vi "9205_Initialize.vi"(7 "Module Model":T1=enum."NI 9205", 8 "error in (no error)":errorcluster, 9 "Slot Settings":T2, 11 "9205 in":refnum<class "9205.lvclass">) -> (0 "error out":errorcluster, 3 "9205 out":refnum<class "9205.lvclass">)   [LabVIEW 2017, in "Modules.lvlib" / "9205.lvclass"]
uses:
  9205.lvclass
  RSI Module/Slot Settings.ctl
  C:/Users/dbuck/Documents/GitHub/Scan-Engine-Custom-Device-Classes/Source/RSI Module/RSI Module.lvclass
  RSI Module/Module Models.ctl
  RSI Module/Channels.ctl
  RSI Module/Channel Type.ctl
  Channel Settings.ctl
  Range.ctl
  Terminal mode.ctl
  9205.lvclass/9205.ctl
  RSI Module/RSI Module.lvclass
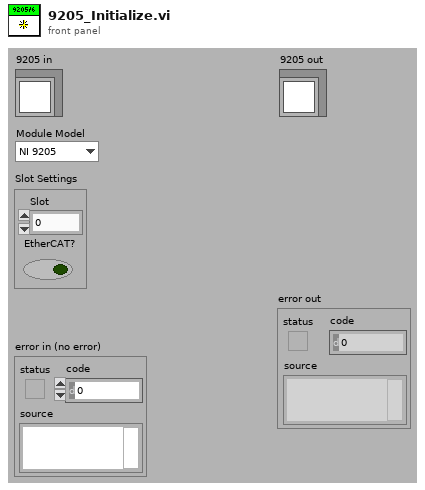
[diagram p1: front panel]
types:
  T1 = typedef "Modules.lvlib/RSI Module.lvclass/Module Models.ctl" = enum16{"Empty", "NI 9201", "NI 9203", "NI 9205", "NI 9206", "NI 9207", "NI 9208", "NI 9211", "NI 9212", "NI 9213", "NI 9214", "NI 9215", "NI 9217", "NI 9219", "NI 9220", "NI 9221", "NI 9222", "NI 9223", "NI 9225", "NI 9227", "NI 9229", "NI 9233", "NI 9234", "NI 9235", "NI 9236", "NI 9237", "NI 9239", "NI 9242", "NI 9244", "NI 9263", "NI 9264", "NI 9265", "NI 9269", "NI 9375", "NI 9401", "NI 9402", "NI 9403", "NI 9411", "NI 9421", "NI 9422", "NI 9423", "NI 9425", "NI 9426", "NI 9435", "NI 9437", "NI 9472", "NI 9474", "NI 9475", "NI 9476", "NI 9477", "NI 9478", "NI 9481", "NI 9482", "NI 9485"}
  T2 = typedef "Modules.lvlib/RSI Module.lvclass/Slot Settings.ctl" = cluster{"Slot":u32, "EtherCAT?":bool}
  T3 = typedef "Modules.lvlib/9205.lvclass/Channel Settings.ctl" = cluster{"Range":T4, "Terminal mode":T5}[]
  T4 = typedef "Modules.lvlib/9205.lvclass/Range.ctl" = u32
  T5 = typedef "Modules.lvlib/9205.lvclass/Terminal mode.ctl" = u32
  T6 = typedef "Modules.lvlib/RSI Module.lvclass/Channels.ctl" = cluster{"# Input Channels":i32, "# Output Channels":i32, "Channel Type":T7, "Units":string}
  T7 = typedef "Modules.lvlib/RSI Module.lvclass/Channel Type.ctl" = enum16{"Analog", "Digital"}
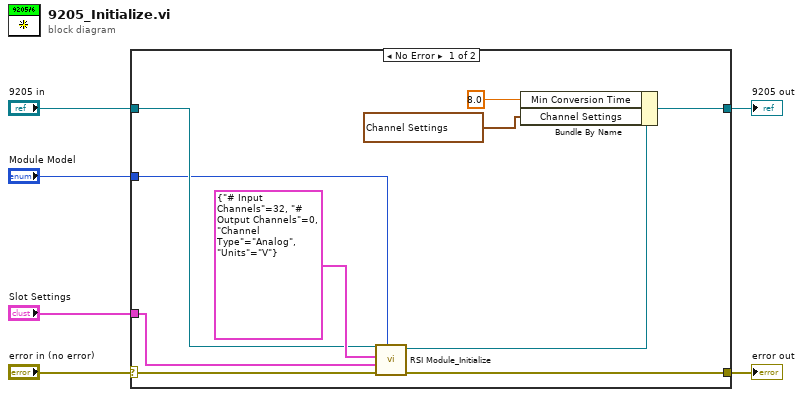
[diagram p0: block diagram]
diagram:
  n1 = case shown="No Error" "error in (no error)" {
    selector: "error in (no error)" -> [w13 w18]
    tunnel: [w9 w18] -> w5
    tunnel: [w10 w17] -> w3
    tunnel: "9205 in" -> [w15 w17]
    tunnel: "Slot Settings" -> [w14 _]
    tunnel: "Module Model" -> [w8 _]
    frame No Error {
      n2 = call "RSI Module_Initialize.vi"("Module Model"=w8, "error in (no error)"=w13, "Slot Settings"=w14, "Channels"=T6 {"# Input Channels"=32, "# Output Channels"=0, "Channel Type"=enum."Analog", "Units"="V"}, "RSI Module in"=w15) -> ("error out"=w9:errorcluster, "RSI Module out"=w12:refnum<class "9205.lvclass">)  [unwired: 5 in]
      n3 = Bundle By Name(cluster=w12, "Min Conversion Time"=8.0 ("Minimum Conversion Time [us]"), "Channel Settings"=T3 [{"Range"=0, "Terminal mode"=0}, {"Range"=0, "Terminal mode"=0}, {"Range"=0, "Terminal mode"=0}, {"Range"=0, "Terminal mode"=0}, {"Range"=0, "Terminal mode"=0}, {"Range"=0, "Terminal mode"=0}, {"Range"=0, "Terminal mode"=0}, {"Range"=0, "Terminal mode"=0}, {"Range"=0, "Terminal mode"=0}, {"Range"=0, "Terminal mode"=0}, {"Range"=0, "Terminal mode"=0}, {"Range"=0, "Terminal mode"=0}, {"Range"=0, "Terminal mode"=0}, {"Range"=0, "Terminal mode"=0}, {"Range"=0, "Terminal mode"=0}, {"Range"=0, "Terminal mode"=0}, {"Range"=0, "Terminal mode"=0}, {"Range"=0, "Terminal mode"=0}, {"Range"=0, "Terminal mode"=0}, {"Range"=0, "Terminal mode"=0}, {"Range"=0, "Terminal mode"=0}, {"Range"=0, "Terminal mode"=0}, {"Range"=0, "Terminal mode"=0}, {"Range"=0, "Terminal mode"=0}, {"Range"=0, "Terminal mode"=0}, {"Range"=0, "Terminal mode"=0}, {"Range"=0, "Terminal mode"=0}, {"Range"=0, "Terminal mode"=0}, {"Range"=0, "Terminal mode"=0}, {"Range"=0, "Terminal mode"=0}, {"Range"=0, "Terminal mode"=0}, {"Range"=0, "Terminal mode"=0}]) -> (w10:refnum<class "9205.lvclass">)
    }
    frame Error {
    }
  }
  "error out" <- w5
  "9205 out" <- w3
